vi "Actor Core.vi"(8 "error in":errorcluster, 11 "Launch IMAQ Display in":refnum<class "HIJ Vision File Viewer App.lvclass">) -> (0 "error out":errorcluster={"status"=FALSE, "code"=0, "source"="Actor Framework.lvlib:Actor.lvclass:Launch Nested Actor.vi<APPEND>\n\n<b>Complete call chain:</b>\r\n     Actor Framework.lvlib:Actor.lvclass:Launch Nested Actor.vi\r\n     Launch HIJ FileViewer.lvlib:Launch File Viewer.lvclass:Actor Core.vi"}, 3 "Actor out":refnum<class "Actor.lvclass">)   [LabVIEW 2014, in "HIJ Vision File Viewer App.lvlib" / "HIJ Vision File Viewer App.lvclass"]
doc: "(<B>Filename</B>: Actor Framework.lvlib:Actor.lvclass:Actor Core.vi)\n\nReceives messages to the actor, reacts to them, and initiates any error handling that may shut the actor down.\n\nDescendant classes may override this VI to append parallel tasks for the actor to complete while it handles messages. Overrides use the Call Parent Method node."
uses:
  HIJ Vision File Viewer App.lvclass
  <vilib>/ActorFramework/Actor/Actor.lvclass
  Display Actors/HIJ Vision File Display/HIJ Vision File Display/HIJ Vision File Display.lvclass
  Analyze/Analyze Classes/Analyze Diviation/Analyze BeamDeviation.lvclass
  Analyze/Results and Overlays/Results Beam Deviation/Analyze Results Beam Deviation.lvclass
  Analyze/Analyze Classes/Analyze Distanz/Analyze Distanz.lvclass
  Analyze/Results and Overlays/Results Distance/Analyze Results Distanz.lvclass
  Analyze/Analyze Classes/Analyze Fluence/Analyze Fluence.lvclass
  Analyze/Results and Overlays/Results Fluence/Analyze Results Fluence.lvclass
  Analyze/Analyze Parameter/Analyze Parameter Energy/Analyze Parameter Energy.lvclass
  Analyze/Analyze Parameter/Analyze Parameter Fluence/Analyze Parameter Fluence.lvclass
  Analyze/Analyze Parameter/Analyze Parameter Energy/Analyze Parameter Energy.lvclass/Analyze Parameter Energy.ctl
  Display Actors/HIJ Vision Display/HIJ Vision Display/HIJ Vision Display.lvclass/HIJ Vision Display.ctl
  HIJ Vision Application/HIJ Vision Application/HIJ Vision Application.lvclass/HIJ Vision Application.ctl
  <vilib>/ActorFramework/Actor/Actor.lvclass/Actor.ctl
  <vilib>/ActorFramework/Message Enqueuer/Message Enqueuer.lvclass/Message Enqueuer.ctl
  Analyze/Results and Overlays/Results Fluence/Analyze Results Fluence.lvclass/Analyze Results Fluence.ctl
  HIJ Vision File Viewer App Messages/Load Image from File Msg/Load Image from File Msg.lvclass/Load Image from File Msg.ctl
  HIJ Vision File Viewer App Messages/Proceed Directory Msg/Proceed Directory Msg.lvclass/Proceed Directory Msg.ctl
  Analyze/Analyze Parameter/Analyze Parameter Energy/Write Energy.vi
  Analyze/Results and Overlays/Results Fluence/Write UI Ref Max F.vi
  Display Actors/HIJ Vision Display/HIJ Vision Display/Write Save Report_.vi
  Display Actors/HIJ Vision Display/HIJ Vision Display/Write Show ZoomBtn_.vi
  HIJ Vision Application/HIJ Vision Application/Write SubPnl for Display.vi
  <vilib>/ActorFramework/Message Enqueuer/Init from Existing Queue.vi
  <vilib>/ActorFramework/Message Enqueuer/Enqueue.vi
  HIJ Vision Application/HIJ Vision Application/Write HIJ Vision Display.vi
  <vilib>/ActorFramework/Message Priority Queue/Priority Enqueue.vi
  <vilib>/ActorFramework/Message Enqueuer/Message Enqueuer.lvclass
  <vilib>/ActorFramework/Stop Msg/Stop Msg.lvclass
  HIJ Vision File Viewer App Messages/Load Image from File Msg/Load Image from File Msg.lvclass
  HIJ Vision File Viewer App Messages/Proceed Directory Msg/Proceed Directory Msg.lvclass
  HIJ Vision Application/HIJ Vision Application/HIJ Vision Application.lvclass
panel:
  in  "Stop Button":bool=TRUE
  in  "Load Image Report":bool=TRUE
  in  "Image File":path=path "C:/Users/user/Desktop/test/WorkDir"
  in  "Proceed Directory":bool
  in  "Previous Image":bool
  in  "Next Image":bool
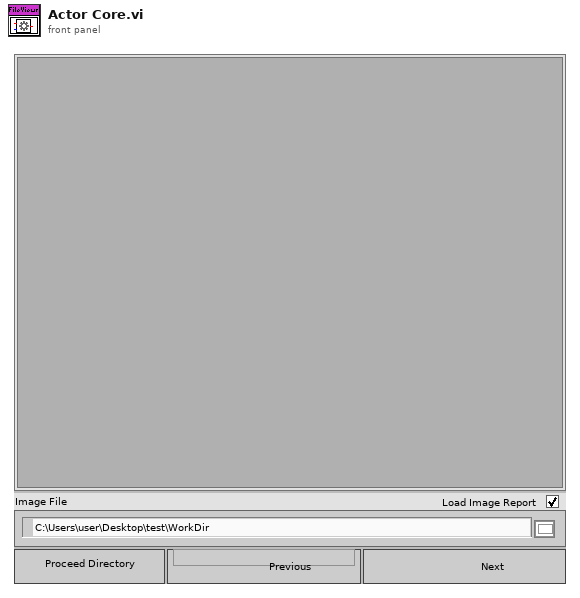
[diagram p1: front panel]
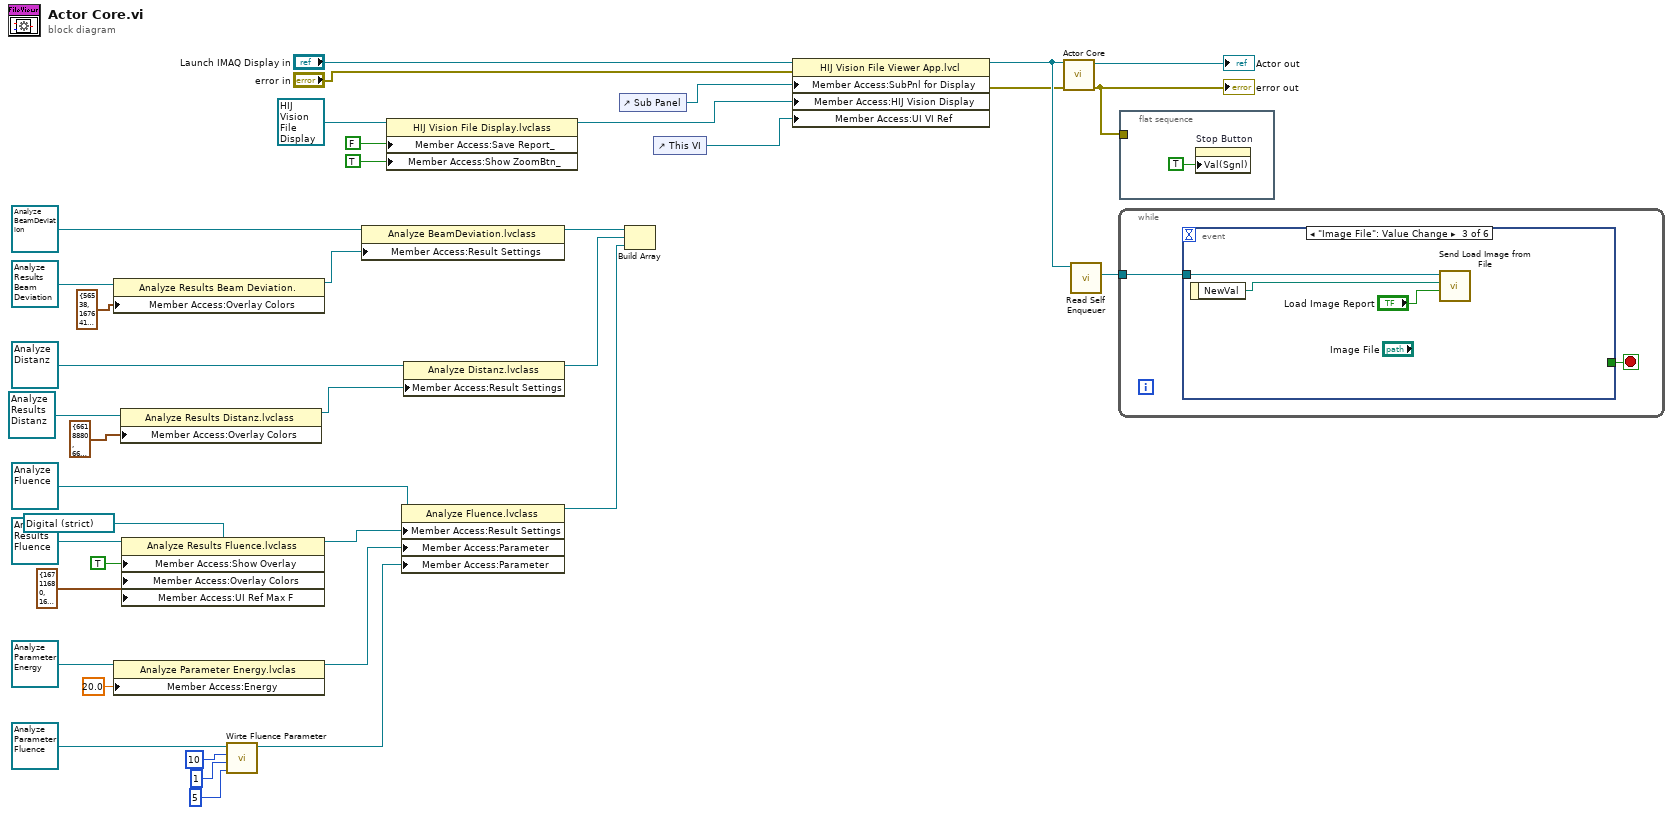
[diagram p0: block diagram]
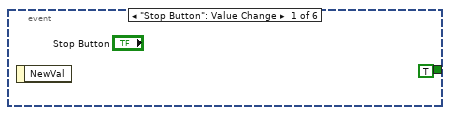
[diagram p2: hidden frame]
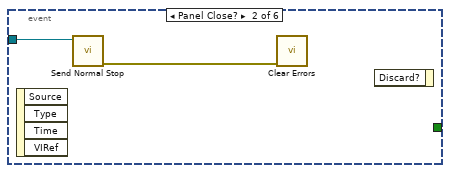
[diagram p3: hidden frame]
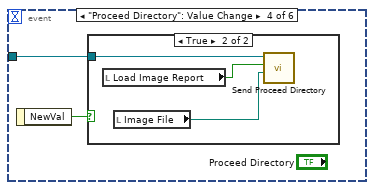
[diagram p4: hidden frame]
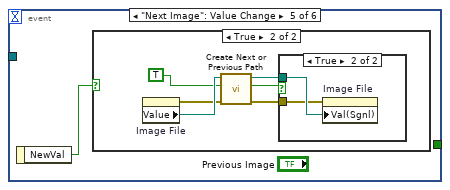
[diagram p6: hidden frame]
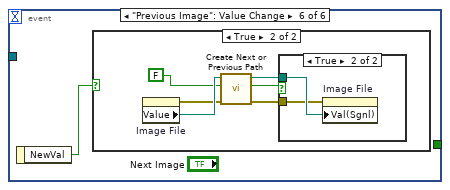
[diagram p9: hidden frame]
diagram:
  n1 = property class="Analyze Results Beam Deviation."(reference=refnum<class "Analyze Results Beam Deviation.lvclass"> refnum ("Analyze Results Beam Deviation.lvclass"), "Member Access:Overlay Colors"=cluster{"Border":u32, "Text":u32} {"Border"=56538, "Text"=16764160} ("Colors")) -> (reference out=w17:refnum<class "Analyze Results Beam Deviation.lvclass">)  [unwired: 1 in, 1 out]
  n2 = property class="Analyze Parameter Energy.lvclas"(reference=refnum<class "Analyze Parameter Energy.lvclass"> refnum ("Analyze Parameter Energy.lvclass"), "Member Access:Energy"=dbl[unit] 20.0 ("Energy")) -> (reference out=w20:refnum<class "Analyze Parameter Energy.lvclass">)  [unwired: 1 in, 1 out]
  n3 = property class="Analyze Results Distanz.lvclass"(reference=refnum<class "Analyze Results Distanz.lvclass"> refnum ("Analyze Results Distanz.lvclass"), "Member Access:Overlay Colors"=cluster{"Border":u32, "Text":u32} {"Border"=6618880, "Text"=6618880} ("Colors")) -> (reference out=w18:refnum<class "Analyze Results Distanz.lvclass">)  [unwired: 1 in, 1 out]
  n4 = property class="Analyze Results Fluence.lvclass"(reference=refnum<class "Analyze Results Fluence.lvclass"> refnum ("Analyze Results Fluence.lvclass"), "Member Access:Show Overlay"=TRUE ("bOverlay"), "Member Access:Overlay Colors"=cluster{"Border":u32, "Text":u32} {"Border"=16711680, "Text"=16448250} ("Colors"), "Member Access:UI Ref Max F"=refnum<vi> refnum ("UI Ref Max F")) -> (reference out=w15:refnum<class "Analyze Results Fluence.lvclass">)  [unwired: 1 in, 1 out]
  n5 = call "Wirte Fluence Parameter.vi"("#of Areas"=5, "#Overlays"=1, "Size of region (px)"=10, "Analyze Parameter Fluence in"=refnum<class "Analyze Parameter Fluence.lvclass"> refnum ("Analyze Parameter Fluence.lvclass")) -> ("Analyze Parameter Fluence out"=w22:refnum<class "Analyze Parameter Fluence.lvclass">)  [unwired: 7 in]
  n6 = property class="Analyze BeamDeviation.lvclass"(reference=refnum<class "Analyze BeamDeviation.lvclass"> refnum ("Analyze.lvlib:Analyze BeamDeviation.lvclass"), "Member Access:Result Settings"=w17) -> (reference out=w16:refnum<class "Analyze BeamDeviation.lvclass">)  [unwired: 1 in, 1 out]
  n7 = property class="HIJ Vision File Display.lvclass"(reference=refnum<class "HIJ Vision File Display.lvclass"> refnum ("HIJ Vision File Viewer.lvlib:HIJ Vision File Viewer.lvclass"), "Member Access:Save Report_"=FALSE ("Save Report_"), "Member Access:Show ZoomBtn_"=TRUE ("Show ZoomBtn_")) -> (reference out=w29:refnum<class "HIJ Vision File Display.lvclass">)  [unwired: 1 in, 1 out]
  n8 = property class="Analyze Fluence.lvclass"(reference=refnum<class "Analyze Fluence.lvclass"> refnum ("Analyze.lvlib:Analyze Fluence.lvclass"), "Member Access:Result Settings"=w15, "Member Access:Parameter"=w20, "Member Access:Parameter"=w22) -> (reference out=w27:refnum<class "Analyze Fluence.lvclass">)  [unwired: 1 in, 1 out]
  n9 = property class="Analyze Distanz.lvclass"(reference=refnum<class "Analyze Distanz.lvclass"> refnum ("Analyze.lvlib:Analyze Distanz.lvclass"), "Member Access:Result Settings"=w18) -> (reference out=w26:refnum<class "Analyze Distanz.lvclass">)  [unwired: 1 in, 1 out]
  n10 = control-ref of="Sub Panel"() -> (w28:refnum<vi>)
  n11 = Build Array(w16, w26, w27) -> ()  [unwired: 1 out]
  n12 = control-ref of="This VI"() -> (w1:refnum<vi>)
  n13 = property class="HIJ Vision File Viewer App.lvcl"(reference="Launch IMAQ Display in", error in="error in", "Member Access:SubPnl for Display"=w28, "Member Access:HIJ Vision Display"=w29, "Member Access:UI VI Ref"=w1) -> (reference out=w31:refnum<class "HIJ Vision File Viewer App.lvclass">, error out=w30:errorcluster)
  n14 = call-parent "Actor Core.vi"("error in"=w30, "HIJ Vision Application in"=w31) -> ("error out"=w37:errorcluster, "Actor out"=→"Actor out":refnum<class "Actor.lvclass">)  [unwired: 8 in]
  "error out" <- w37
  n15 = call <vilib>:"Read Self Enqueuer.vi"("Actor"=w31) -> ("Self Enqueuer"=w36:refnum<class "Message Enqueuer.lvclass">)  [unwired: 10 in]
  n16 = while {
    tunnel: w36 -> [w39]
    stop <- w40 stop-if-true
    n17 = event shown="[2] \"Image File\": Value Change" {
      selector: _ -> [_ _ _ _ _ _]
      dyn-events: _ -> [_ _ _ _ _ _]
      timeout: _ -> [_ _ _ _ _ _]
      tunnel: [TRUE _ _ _ _ _] -> w40
      tunnel: w39 -> [_ w43 w46 w47 _ _]
      event "Stop Button": Value Change {
        n18 = event-data() -> ()  [unwired: 1 in, 1 out]
      }
      event Panel Close? {
        n19 = event-data() -> ()  [unwired: 1 in, 4 out]
        n20 = call <vilib>:"Send Normal Stop.vi"("Message Enqueuer"=w43) -> ("error out"=w42:errorcluster)  [unwired: 10 in]
        n21 = call <vilib>:"Clear Errors.vi"("error in (no error)"=w42) -> ()  [unwired: 5 in, 2 out]
        n22 = event-data() -> ()  [unwired: 2 in, 1 out]
      }
      event "Image File": Value Change {
        n23 = event-data() -> ("NewVal"=w45:path)  [unwired: 1 in]
        n24 = call "Send Load Image from File.vi"("Load Report"="Load Image Report", "Image"=w45, "Message Enqueuer"=w46) -> ()  [unwired: 7 in, 2 out]
      }
      event "Proceed Directory": Value Change {
        n25 = event-data() -> ("NewVal"=w48:bool)  [unwired: 1 in]
        n26 = case shown="True" w48 {
          tunnel: w47 -> [_ w51]
          frame False {
          }
          frame True {
            n27 = local read "Load Image Report"() -> (w49:bool)
            n28 = local read "Image File"() -> (w50:path)
            n29 = call "Send Proceed Directory.vi"("path"=w50, "Load Image Report"=w49, "Message Enqueuer"=w51) -> ()  [unwired: 7 in, 2 out]
          }
        }
      }
      event "Next Image": Value Change {
        n30 = event-data() -> ("NewVal"=w52:bool)  [unwired: 1 in]
        n31 = case shown="True" w52 {
          frame False {
          }
          frame True {
            n32 = property on="Image File" class="Path"() -> (error out=w57:errorcluster, "Value"=w58:path)  [unwired: 2 in, 1 out]
            n33 = call "Create Next or Previous Path.vi"("error in (no error)"=w57, "Next?"=TRUE, "current image"=w58) -> ("error out"=w55:errorcluster, "file or folder exists?"=w54:bool, "next or previous image"=w56:path)  [unwired: 6 in]
            n34 = case shown="True" w54 {
              tunnel: w56 -> [_ w60]
              tunnel: w55 -> [_ w59]
              frame False {
              }
              frame True {
                n35 = property on="Image File" class="Path"(error in=w59, "Val(Sgnl)"=w60) -> ()  [unwired: 1 in, 2 out]
              }
            }
          }
        }
      }
      event "Previous Image": Value Change {
        n36 = event-data() -> ("NewVal"=w61:bool)  [unwired: 1 in]
        n37 = case shown="True" w61 {
          frame False {
          }
          frame True {
            n38 = property on="Image File" class="Path"() -> (error out=w66:errorcluster, "Value"=w67:path)  [unwired: 2 in, 1 out]
            n39 = call "Create Next or Previous Path.vi"("error in (no error)"=w66, "Next?"=FALSE, "current image"=w67) -> ("error out"=w64:errorcluster, "file or folder exists?"=w63:bool, "next or previous image"=w65:path)  [unwired: 6 in]
            n40 = case shown="True" w63 {
              tunnel: w65 -> [_ w69]
              tunnel: w64 -> [_ w68]
              frame False {
              }
              frame True {
                n41 = property on="Image File" class="Path"(error in=w68, "Val(Sgnl)"=w69) -> ()  [unwired: 1 in, 2 out]
              }
            }
          }
        }
      }
    }
  }
  n42 = flat-sequence {
    tunnel: w37 -> [_]
    frame #0 {
      n43 = property on="Stop Button" class="Bool (strict)"("Val(Sgnl)"=TRUE) -> ()  [unwired: 2 in, 2 out]
    }
  }
